vi "Peek Raw Socket.vi"(8 "error in (no error)":errorcluster, 10 "socket":u64) -> (0 "error out":errorcluster, 1 "buffer":string, 2 "bytes waiting":i32)   [LabVIEW 2015, in "Win32 Util.lvlib"]
uses:
  LabSDL2/Source/Libraries/Win32 Util/Win32 Util.lvlib
  wsock32.dll
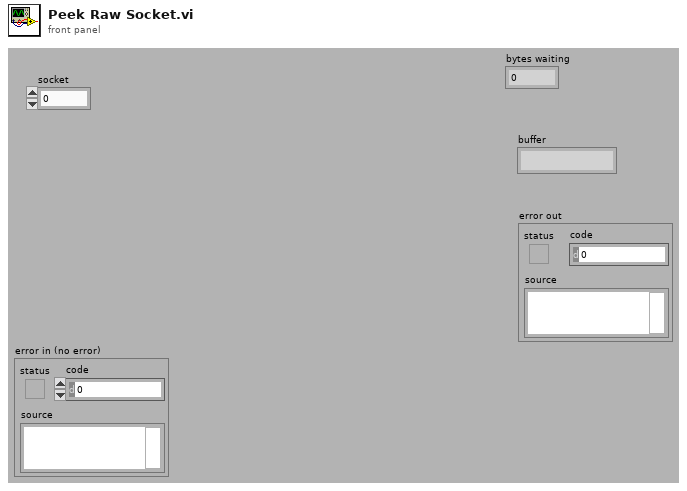
[diagram p1: front panel]
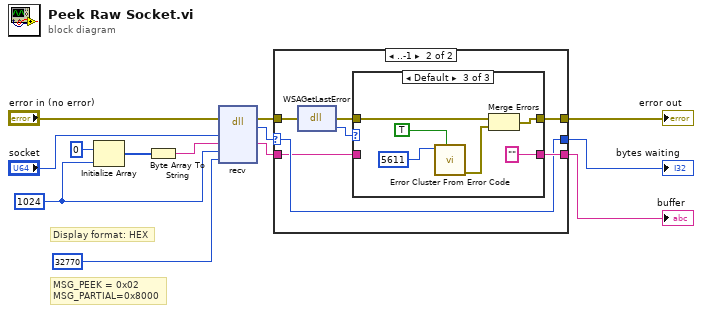
[diagram p0: block diagram]
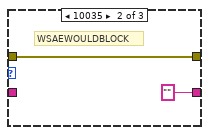
[diagram p4: hidden frame]
diagram:
  w4 = 1024 ("len")
  # "Display format: HEX"
  # "MSG_PEEK = 0x02\nMSG_PARTIAL=0x8000"
  n1 = Initialize Array(u8 0 ("element"), w4) -> (w2:u8[])
  n2 = Byte Array To String(unsigned byte array=w2) -> (string=w1:string)
  n3 = dll-call lib="wsock32.dll" fn="recv"(error in="error in (no error)", "socket"="socket", "buffer"=w1, "len"=w4, "flags"=u32 32770) -> (error out=w6:errorcluster, "return type"=w10:i32, "buffer"=w8:string)  [unwired: 5 in, 1 out]
  n4 = case shown="..-1" w10 {
    selector: w10 -> [w15 w22]
    tunnel: [w16 w23] -> w9
    tunnel: w8 -> [w16 w18]
    tunnel: [w15 w22] -> w7
    tunnel: [w14 w21] -> w5
    tunnel: w6 -> [w14 w17]
    frame 0.. {
    }
    frame ..-1 {
      n5 = dll-call lib="wsock32.dll" fn="WSAGetLastError"(error in=w17) -> (error out=w20:errorcluster, "return type"=w19:i32)  [unwired: 2 in, 1 out]
      n6 = case shown="Default" w19 {
        tunnel: [w24 "" ("buffer") "" ("buffer")] -> w23
        tunnel: [w25 w27 w29] -> w21
        tunnel: w20 -> [w25 w27 w28]
        tunnel: w18 -> [w24 _ _]
        frame 10040 {
          # "WSAEMSGSIZE"
        }
        frame 10035 {
          # "WSAEWOULDBLOCK"
        }
        frame Default {
          n7 = call <vilib>:"Error Cluster From Error Code.vi"("show call chain? (False)"=TRUE, "error code (0)"=5611) -> ("error out"=w30:errorcluster)  [unwired: 7 in]
          n8 = Merge Errors(w28, w30) -> (w29:errorcluster)
        }
      }
    }
  }
  "buffer" <- w9
  "bytes waiting" <- w7
  "error out" <- w5
